vi "Configure Channel.vi"(5 "Vertical Offset (0.0 V)":dbl, 6 "Probe Attenuation (1.0)":dbl=1.0, 7 "Enable Channel (T: Enable)":bool=TRUE, 8 "error in (no error)":errorcluster, 9 "Vertical Range (2.0 V)":dbl=2.0, 10 "Channel (1: Channel 1)":i32(ring)=1 items=["Channel 1"=1, "Channel 2"=2, "Channel 3"=3, "Channel 4"=4], 11 "VISA resource name":refnum<visa-resource-name>) -> (0 "error out":errorcluster, 3 "VISA resource name out":refnum<visa-resource-name>)   [LabVIEW 2020, in "Agilent 90000 Series.lvlib"]
doc: "Configures the common properties of the vertical subsystem of the oscilloscope for the specified channel. Call this VI for each channel you want to enable to acquire waveforms.\n\n<B>Note:</B>\nThe channel settings will not be applied if the channel is not enabled."
uses:
  Agilent 90000 Series.lvlib
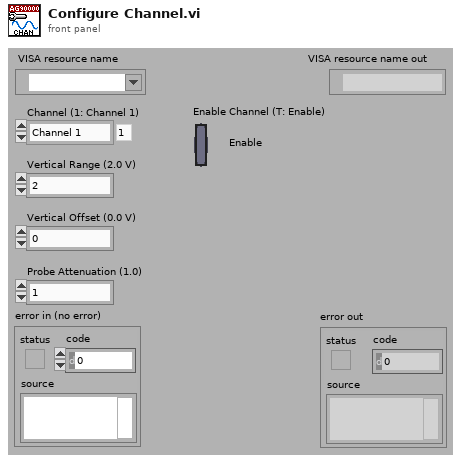
[diagram p1: front panel]
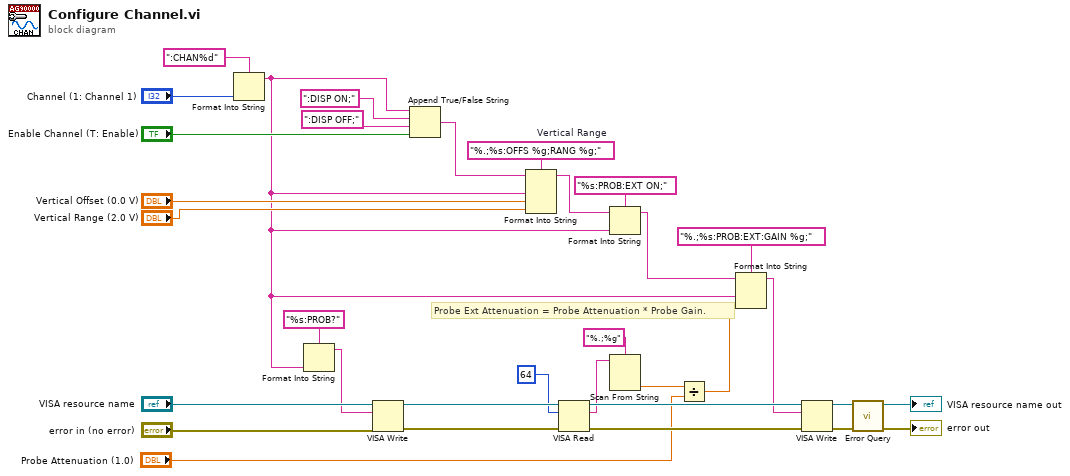
[diagram p0: block diagram]
diagram:
  w21 = "%.;%s:OFFS %g;RANG %g;"  # Vertical Range
  # "Probe Ext Attenuation = Probe Attenuation * Probe Gain."
  n1 = Format Into String(format string=":CHAN%d", "Channel (1: Channel 1)") -> (resulting string=w3:string)  [unwired: 2 in, 1 out]
  n2 = Format Into String(format string="%s:PROB?", w3) -> (resulting string=w19:string)  [unwired: 2 in, 1 out]
  n3 = VISA Write(VISA resource name="VISA resource name", write buffer=w19, error in (no error)="error in (no error)") -> (VISA resource name out=w18:refnum<visa-resource-name>, error out=w17:errorcluster)  [unwired: 1 out]
  n4 = Append True/False String(1:"Enable Channel (T: Enable)", 2:":DISP OFF;" ("false string"), 3:":DISP ON;" ("true string"), 4:w3) -> (0:w1:string)
  n5 = Format Into String(format string=w21, initial string=w1, w3, "Vertical Offset (0.0 V)", "Vertical Range (2.0 V)") -> (resulting string=w10:string)  [unwired: 1 in, 1 out]
  n6 = VISA Read(VISA resource name=w18, byte count=u32 64, error in (no error)=w17) -> (VISA resource name out=w27:refnum<visa-resource-name>, read buffer=w15:string, error out=w26:errorcluster)  [unwired: 1 out]
  n7 = Format Into String(format string="%s:PROB:EXT ON;", initial string=w10, w3) -> (resulting string=w8:string)  [unwired: 1 in, 1 out]
  n8 = Scan From String(format string="%.;%g", input string=w15) -> (output 1=w12:dbl)  [unwired: 2 in, 4 out]
  n9 = Divide(x=w12, y="Probe Attenuation (1.0)") -> (x/y=w13:dbl)
  n10 = Format Into String(format string="%.;%s:PROB:EXT:GAIN %g;", initial string=w8, w3, w13) -> (resulting string=w6:string)  [unwired: 1 in, 1 out]
  n11 = VISA Write(VISA resource name=w27, write buffer=w6, error in (no error)=w26) -> (VISA resource name out=w31:refnum<visa-resource-name>, error out=w30:errorcluster)  [unwired: 1 out]
  n12 = call "Error Query.vi"("error in (no error)"=w30, "VISA resource name"=w31) -> ("error out"=→"error out":errorcluster, "VISA resource name out"=→"VISA resource name out":refnum<visa-resource-name>)  [unwired: 8 out]
